vi "niRFUtil WFM Align Waveforms - Fine (real wfm).vi"(0 "Waveform In":T2 {"y" min=0 max=127 format="%.2f"; "dx" format="%^.2e"; "x0" format="%^.2e"}, 5 "Reference Waveform":T2 {"y" min=0 max=127 format="%.2f"; "dx" format="%^.2e"; "x0" format="%^.2e"}, 7 "Filter Phase Estimates":T1=enum."True", 9 "Filter Length (samples)":i32=20, 13 "Flush Buffers?":bool) -> (4 "Waveform Out":T2 {"y" min=0 max=127 format="%.2f"; "dx" format="%^.2e"; "x0" format="%^.2e"})   [LabVIEW 2015, in "niRFUtil.lvlib"]
doc: "(c) Copyright 2006, National Instruments, Inc. This VI may not be duplicated, sold, or distributed without written consent from National Instruments."
uses:
  niRFUtil.lvlib
  Includes/niRFUtil INC Real Waveform.ctl
  Includes/niRFUtil INC Real Array.ctl
  Includes/niRFUtil INC Filter Phase Estimates.ctl
  niRFUtil WFM Moving Average (complex array).vi
  Filters, Transforms, Windows/niRFUtil FTW FFT (complex wfm).vi
  niRFUtil WFM Complex Differential (complex wfm).vi
  niRFUtil WFM Parse Waveform - Duration (real wfm).vi
  Measurements/niRFUtil MEAS Waveform Statistics (real wfm).vi
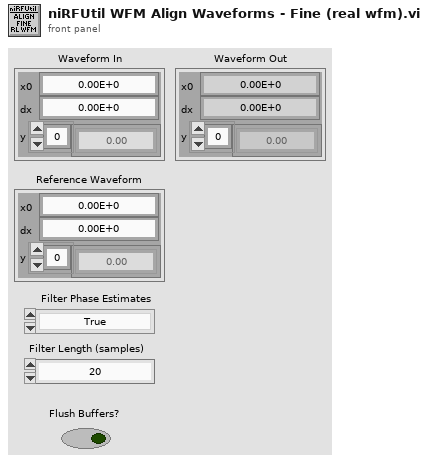
[diagram p1: front panel]
types:
  T1 = typedef "niRFUtil.lvlib/niRFUtil INC Filter Phase Estimates.ctl" = enum16{"False", "True"}
  T2 = typedef "niRFUtil.lvlib/niRFUtil INC Real Waveform.ctl" = cluster{"x0":dbl, "dx":dbl, "y":T3}
  T3 = typedef "niRFUtil.lvlib/niRFUtil INC Real Array.ctl" = sgl[]
  T4 = typedef "niRFUtil.lvlib/niRFUtil INC Complex Waveform.ctl" = cluster{"x0":dbl, "dx":dbl, "y":T5}
  T5 = typedef "niRFUtil.lvlib/niRFUtil INC Complex Array.ctl" = csg[]
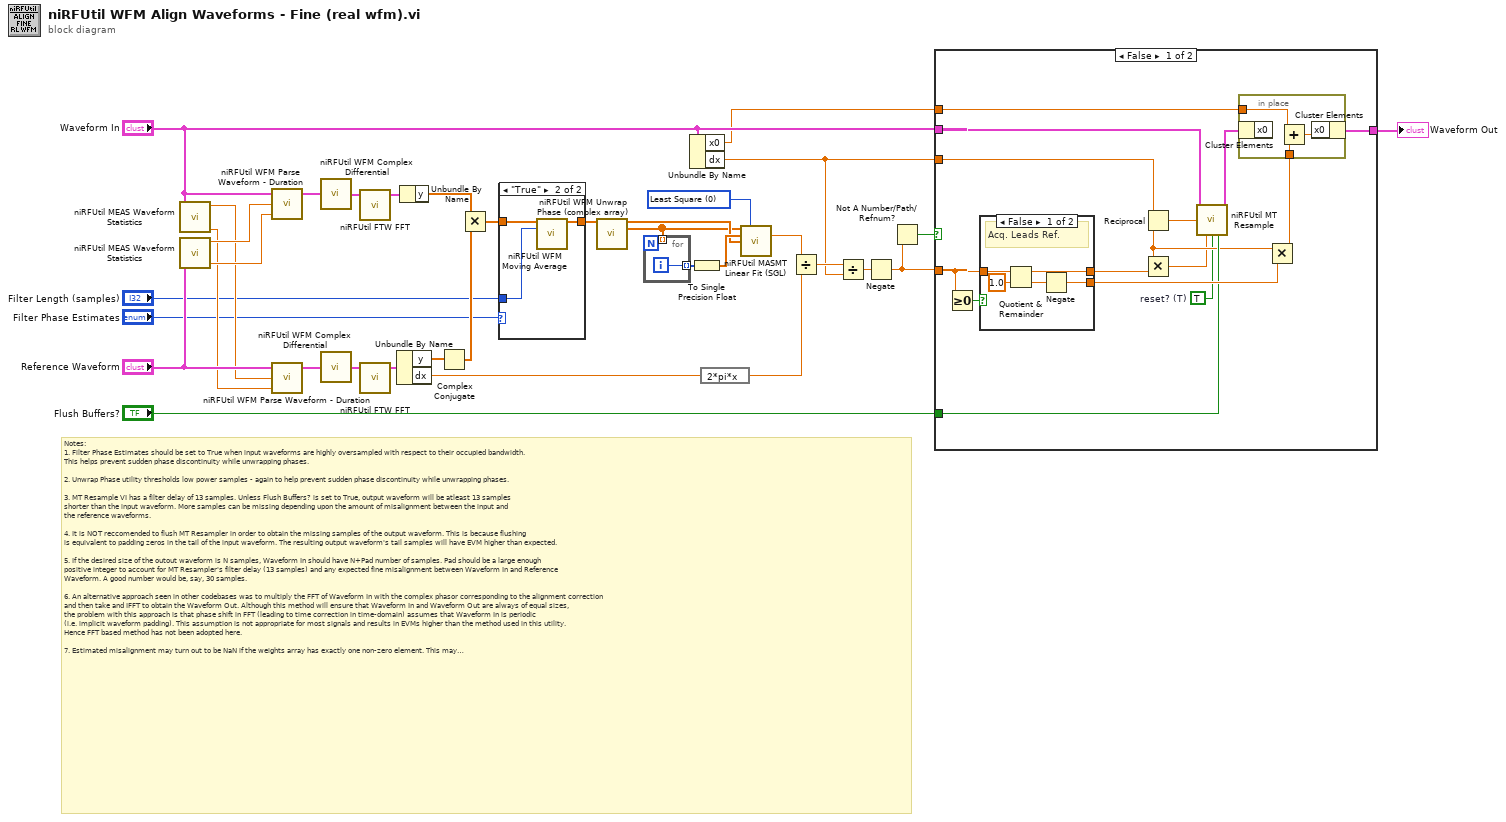
[diagram p0: block diagram]
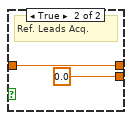
[diagram p2: hidden frame]
diagram:
  w26 = 0 items=["Least Square", "Least Absolute Residual", "Bisquare"] ("method")
  # "Notes:\n1. Filter Phase Estimates should be set to True when input waveforms are highly oversampled with respect to their occupied bandwidth. \nThis helps prevent sudden phase discontinuity while unwrapping phases.\n\n2. Unwrap Phase utility thresholds low power samples - again to help prevent sudden phase discontinuity while unwrapping phases.\n\n3. MT Resample VI has a filter delay of 13 samples. Unless Flush Buffers? is set to True, output waveform will be atleast 13 samples \nshorter than the input waveform. More samples can be missing depending upon the amount of misalignment between the input and\nthe reference waveforms.\n\n4. It is NOT reccomended to flush MT Resampler in order to obtain the missing samples of the output waveform. This is because flushing\nis equivalent to padding zeros in the tail of the input waveform. The resulting output waveform's tail samples will have EVM higher than expected.\n\n5. If the desired size of the outout waveform is N samples, Waveform In should have N+Pad number of samples. Pad should be a large enough \npositive integer to account for MT Resampler's filter delay (13 samples) and any expected fine misalignment between Waveform In and Reference\nWaveform. A good number would be, say, 30 samples.\n\n6. An alternative approach seen in other codebases was to multiply the FFT of Waveform In with the complex phasor corresponding to the alignment correction\nand then take and IFFT to obtain the Waveform Out. Although this method will ensure that Waveform In and Waveform Out are always of equal sizes,\nthe problem with this approach is that phase shift in FFT (leading to time correction in time-domain) assumes that Waveform In is periodic \n(i.e. implicit waveform padding). This assumption is not appropriate for most signals and results in EVMs higher than the method used in this utility.\nHence FFT based method has not been adopted here.\n\n7. Estimated misalignment may turn out to be NaN if the weights array has exactly one non-zero element. This may happen with sinusoids. \nIn that case, no correction is done."
  n1 = call-poly "niRFUtil MEAS Waveform Statistics.vi"("Waveform In"="Waveform In") -> ("Start"=w19:dbl, "Duration"=w18:dbl)  [unwired: 6 out]
  n2 = call-poly "niRFUtil MEAS Waveform Statistics.vi"("Waveform In"="Reference Waveform") -> ("Start"=w20:dbl, "Duration"=w21:dbl)  [unwired: 6 out]
  n3 = call-poly "niRFUtil WFM Parse Waveform - Duration.vi"("Duration (Inf)"=w21, "Start (-Inf)"=w20, "Waveform In"="Waveform In") -> ("Waveform Out"=w24:T2)  [unwired: 2 out]
  n4 = call-poly "niRFUtil WFM Parse Waveform - Duration.vi"("Duration (Inf)"=w18, "Start (-Inf)"=w19, "Waveform In"="Reference Waveform") -> ("Waveform Out"=w22:T2)  [unwired: 2 out]
  n5 = call-poly "niRFUtil WFM Complex Differential.vi"("Waveform In"=w24) -> ("Waveform Out"=w25:T4)  [unwired: 14 out]
  n6 = call-poly "niRFUtil WFM Complex Differential.vi"("Waveform In"=w22) -> ("Waveform Out"=w35:T4)  [unwired: 14 out]
  n7 = call-poly "niRFUtil FTW FFT.vi"("Waveform In (V)"=w25) -> ("Waveform Out (V)"=w34:T4)  [unwired: 2 in, 2 out]
  n8 = call-poly "niRFUtil FTW FFT.vi"("Waveform In (V)"=w35) -> ("Waveform Out (V)"=w33:T4)  [unwired: 2 in, 2 out]
  n9 = Unbundle By Name(w33) -> ("y"=w13:T5, "dx"=w31:dbl)
  n10 = Unbundle By Name(w34) -> ("y"=w16:T5)
  n11 = Complex Conjugate(1:w13) -> (0:w17:T5)
  n12 = Multiply(x=w16, y=w17) -> (x*y=w15:T5)
  n13 = case shown="\"True\"" "Filter Phase Estimates" {
    tunnel: w15 -> [w36 w39]
    tunnel: [w36 w38] -> w12
    tunnel: "Filter Length (samples)" -> [_ w37]
    frame "False" {
    }
    frame "True" {
      n14 = call-poly "niRFUtil WFM Moving Average.vi"("Array In"=w39, "Averaging Window (samples)"=w37) -> ("Averaged Array Out"=w38:T5)  [unwired: 13 in]
    }
  }
  n15 = call "niRFUtil WFM Unwrap Phase (complex array).vi"("Complex Vectors"=w12) -> ("Magnitude"=w11:T3, "Unwrapped Phase (rad)"=w10:T3)  [unwired: 13 in]
  n16 = for {
    tunnel: w10 -> [_] mode=indexing
    tunnel: [w40] -> w32 mode=indexing
    i -> [w40]
  }
  n17 = Unbundle By Name("Waveform In") -> ("x0"=w1:dbl, "dx"=w4:dbl)
  n18 = To Single Precision Float(number=w32) -> (single precision float=w14:sgl[])
  n19 = expression code="2*pi*x"(w31) -> (w29:dbl)
  n20 = call "niRFUtil MASMT Linear Fit (SGL).vi"("Y"=w10, "method"=w26, "X"=w14, "Weight"=w11) -> ("slope"=w30:sgl)  [unwired: 7 in, 4 out]
  n21 = Divide(x=w30, y=w29) -> (x/y=w28:dbl)
  n22 = Divide(x=w28, y=w4) -> (x/y=w27:dbl)
  n23 = Negate(x=w27) -> (-x=w3:dbl)
  n24 = Not A Number/Path/Refnum?(number/path/refnum=w3) -> (NaN/Path/Refnum?=w5:bool)
  n25 = case shown="False" w5 {
    tunnel: w3 -> [w47 _]
    tunnel: [w54 w65] -> w2
    tunnel: "Waveform In" -> [w53 w65]
    tunnel: "Flush Buffers?" -> [w49 _]
    tunnel: w4 -> [w48 _]
    tunnel: w1 -> [w46 _]
    frame False {
      w45 = TRUE  # reset? (T)
      n26 = Greater Or Equal To 0?(x=w47) -> (x >= 0?=w52:bool)
      n27 = case shown="False" w52 {
        tunnel: [w58 0.0] -> w51
        tunnel: w47 -> [w62 w64]
        tunnel: [w59 w64] -> w50
        frame False {
          # "Acq. Leads Ref."
          n28 = Quotient & Remainder(x=w62, y=1.0) -> (x-y*floor(x/y)=w59:dbl, floor(x/y)=w60:dbl)
          n29 = Negate(x=w60) -> (-x=w58:dbl)
        }
        frame True {
          # "Ref. Leads Acq."
        }
      }
      n30 = Reciprocal(x=w48) -> (1/x=w44:dbl)
      n31 = Multiply(x=w48, y=w50) -> (x*y=w43:dbl)
      n32 = call "niRFUtil MT Resample.vi"("Waveform In"=w53, "initial sample offset (sec)"=w43, "desired sample rate (Hz)"=w44, "reset? (T)"=w45, "flush buffers? (F)"=w49) -> ("Waveform Out"=w42:T4)  [unwired: 9 in, 1 out]
      n33 = Multiply(x=w48, y=w51) -> (x*y=w41:dbl)
      n34 = in-place {
        in-place-border: w41 -> [w56]
        in-place-border: w46 -> [w55]
        n35 = in-place-cluster #1(w42) -> ()  [unwired: 1 out]
        n36 = Add(x=w55, y=w56) -> (x+y=w57:dbl)
        n37 = in-place-cluster #1("x0"=w57) -> (w54:T4)
      }
    }
    frame True {
    }
  }
  "Waveform Out" <- w2
